vi "GPS_Pos.vi"(8 "error in (no error)":errorcluster, 11 "System Data":T1={"System"={"Active"=FALSE, "Exit"=FALSE, "Command wait"="", "Status_Time"=0, "Time_GPS"=0}, "Stepper Motor"={"Connection Reference"="", "Valid Connection"=FALSE, "Speed"=15}, "Camera Data"={"Image path"=path "", "Filenames"=[], "Filenames queue"=[]}, "Core"={"Close Panel on Exit?"=FALSE, "Current VI Reference"=refnum}} {"Stepper Motor"."Speed" scale=0.0..30.0}) -> (0 "error out":errorcluster, 3 "System Data out":T1={"System"={"Active"=FALSE, "Exit"=FALSE, "Command wait"="", "Status_Time"=0, "Time_GPS"=0}, "Stepper Motor"={"Connection Reference"="", "Valid Connection"=FALSE, "Speed"=15}, "Camera Data"={"Image path"=path "", "Filenames"=[], "Filenames queue"=[]}, "Core"={"Close Panel on Exit?"=FALSE, "Current VI Reference"=refnum}} {"Stepper Motor"."Speed" scale=0.0..30.0})   [LabVIEW 2019]
uses:
  System Data.ctl
  Stepper Data.ctl
  Camera Data.ctl
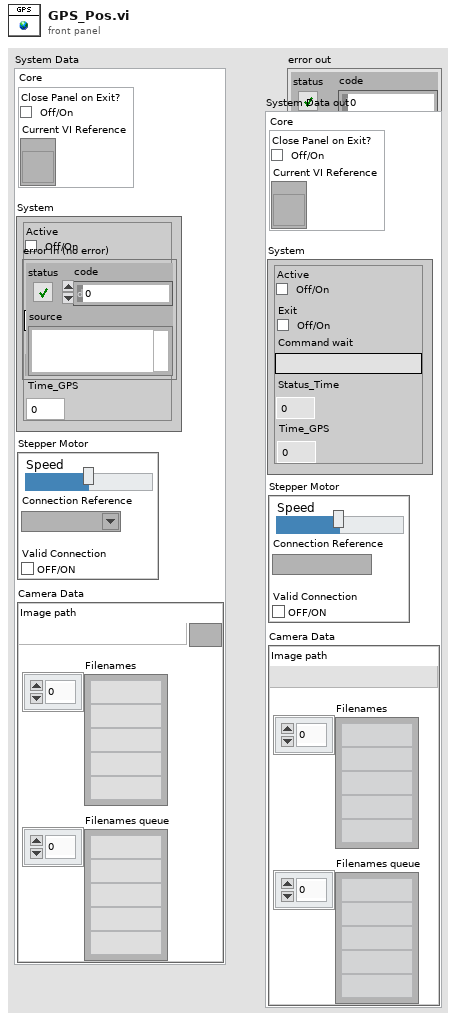
[diagram p1: front panel]
types:
  T1 = typedef "System Data.ctl" = cluster{"System":cluster{"Active":bool, "Exit":bool, "Command wait":string, "Status_Time":i32, "Time_GPS":i32}, "Stepper Motor":T2, "Camera Data":T3, "Core":cluster{"Close Panel on Exit?":bool, "Current VI Reference":refnum<vi>}}
  T2 = typedef "Stepper Data.ctl" = cluster{"Connection Reference":refnum<visa-resource-name>, "Valid Connection":bool, "Speed":i32}
  T3 = typedef "Camera Data.ctl" = cluster{"Image path":path, "Filenames":string[], "Filenames queue":string[]}
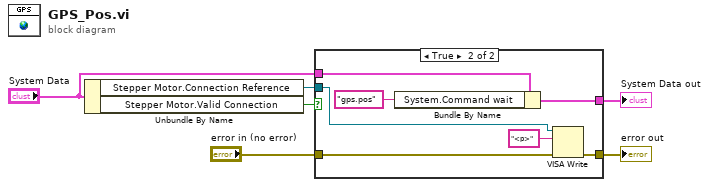
[diagram p0: block diagram]
diagram:
  n1 = Unbundle By Name("System Data") -> ("Stepper Motor.Connection Reference"=w6:refnum<visa-resource-name>, "Stepper Motor.Valid Connection"=w4:bool)
  n2 = case shown="True" w4 {
    tunnel: w6 -> [_ w14]
    tunnel: [w8 w12] -> w5
    tunnel: "error in (no error)" -> [w8 w13]
    tunnel: "System Data" -> [w7 w11]
    tunnel: [w7 w9] -> w1
    frame False {
    }
    frame True {
      n3 = Bundle By Name(cluster=w11, "System.Command wait"="gps.pos") -> (w9:T1)
      n4 = VISA Write(VISA resource name=w14, write buffer="<p>", error in (no error)=w13) -> (error out=w12:errorcluster)  [unwired: 2 out]
    }
  }
  "error out" <- w5
  "System Data out" <- w1
